vi "Set BlowerHeater.vi"(7 "Blower/Heater":T1, 8 "error in (no error)":errorcluster, 10 "ON/OFF (OFF)":bool, 11 "cRIO-CO2 in":refnum<class "cRIO-CO2.lvclass">) -> (0 "error out":errorcluster, 3 "cRIO-CO2 out":refnum<class "cRIO-CO2.lvclass">)   [LabVIEW 2015, in "cRIO-Carbondioxide.lvlib" / "cRIO-CO2.lvlib" / "cRIO-CO2.lvclass"]
uses:
  cRIO-CO2.lvclass
  Blowers Heaters Enumerator.ctl
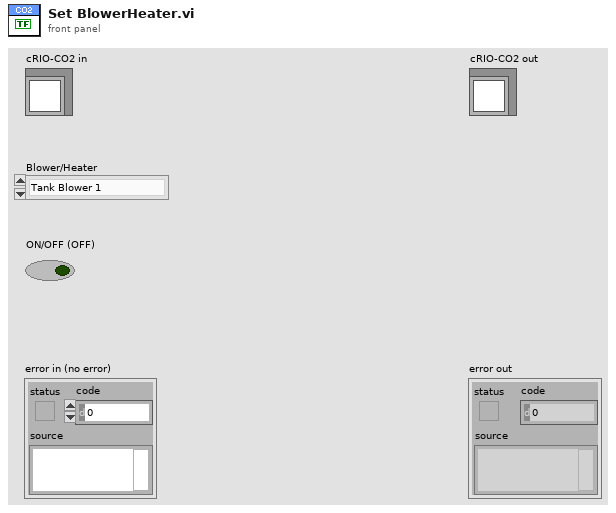
[diagram p1: front panel]
types:
  T1 = typedef "cRIO-Carbondioxide.lvlib/cRIO-CO2.lvlib/cRIO-CO2.lvclass/Blowers Heaters Enumerator.ctl" = enum16{"Tank Blower 1", "Tank Blower 2", "Tank Blower 3", "Tank Blower 4", "Syringe Blower", "Syringe Heater", "Piston Heater", "Undefined"}
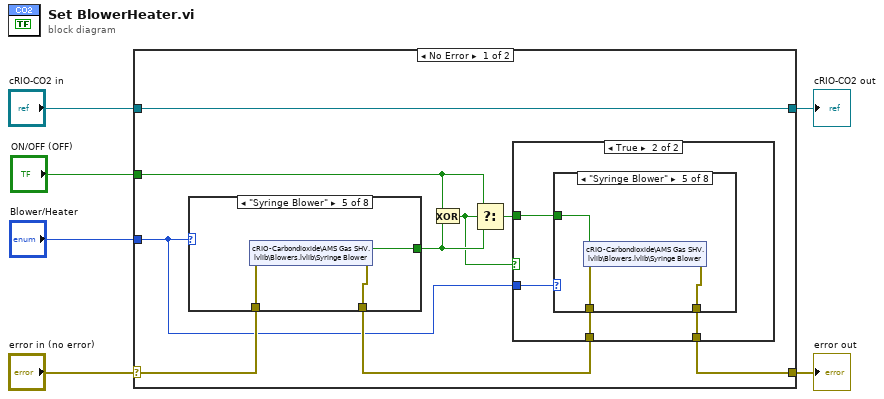
[diagram p0: block diagram]
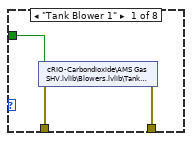
[diagram p3: hidden frame]
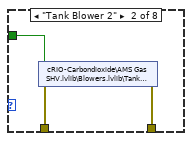
[diagram p4: hidden frame]
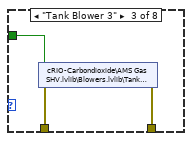
[diagram p5: hidden frame]
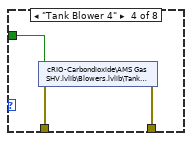
[diagram p6: hidden frame]
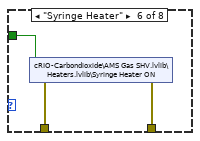
[diagram p7: hidden frame]
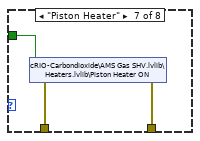
[diagram p8: hidden frame]
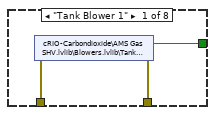
[diagram p10: hidden frame]
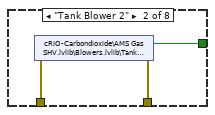
[diagram p11: hidden frame]
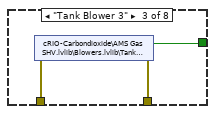
[diagram p12: hidden frame]
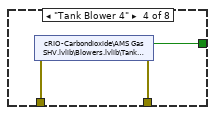
[diagram p13: hidden frame]
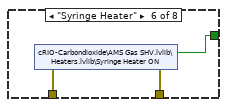
[diagram p14: hidden frame]
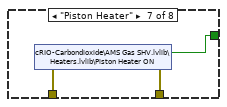
[diagram p15: hidden frame]
diagram:
  n1 = case shown="No Error" "error in (no error)" {
    selector: "error in (no error)" -> [w14 w66]
    tunnel: [w12 w66] -> w5
    tunnel: [w15 w65] -> w3
    tunnel: "cRIO-CO2 in" -> [w15 w65]
    tunnel: "Blower/Heater" -> [w11 _]
    tunnel: "ON/OFF (OFF)" -> [w9 _]
    frame No Error {
      n2 = case shown="\"Syringe Blower\"" w11 {
        tunnel: w14 -> [w45 w48 w51 w54 w57 w60 w63 w64]
        tunnel: [w44 w47 w50 w53 w56 w59 w62 w64] -> w13
        tunnel: [w43 w46 w49 w52 w55 w58 w61 _] -> w10
        frame "Tank Blower 1" {
          n3 = shared-variable "cRIO-Carbondioxide\\AMS Gas SHV.lvlib\\Blowers.lvlib\\Tank Blower 1"(error in=w45) -> (w43:bool, error out=w44:errorcluster)
        }
        frame "Tank Blower 2" {
          n4 = shared-variable "cRIO-Carbondioxide\\AMS Gas SHV.lvlib\\Blowers.lvlib\\Tank Blower 2"(error in=w48) -> (w46:bool, error out=w47:errorcluster)
        }
        frame "Tank Blower 3" {
          n5 = shared-variable "cRIO-Carbondioxide\\AMS Gas SHV.lvlib\\Blowers.lvlib\\Tank Blower 3"(error in=w51) -> (w49:bool, error out=w50:errorcluster)
        }
        frame "Tank Blower 4" {
          n6 = shared-variable "cRIO-Carbondioxide\\AMS Gas SHV.lvlib\\Blowers.lvlib\\Tank Blower 4"(error in=w54) -> (w52:bool, error out=w53:errorcluster)
        }
        frame "Syringe Blower" {
          n7 = shared-variable "cRIO-Carbondioxide\\AMS Gas SHV.lvlib\\Blowers.lvlib\\Syringe Blower"(error in=w57) -> (w55:bool, error out=w56:errorcluster)
        }
        frame "Syringe Heater" {
          n8 = shared-variable "cRIO-Carbondioxide\\AMS Gas SHV.lvlib\\Heaters.lvlib\\Syringe Heater ON"(error in=w60) -> (w58:bool, error out=w59:errorcluster)
        }
        frame "Piston Heater" {
          n9 = shared-variable "cRIO-Carbondioxide\\AMS Gas SHV.lvlib\\Heaters.lvlib\\Piston Heater ON"(error in=w63) -> (w61:bool, error out=w62:errorcluster)
        }
        frame "Undefined" {
        }
      }
      n10 = Exclusive Or(1:w10, 2:w9) -> (0:w7:bool)
      n11 = Select(t=w9, s=w7, f=w10) -> (s? t:f=w8:bool)
      n12 = case shown="True" w7 {
        tunnel: w13 -> [w16 w20]
        tunnel: [w16 w19] -> w12
        tunnel: w11 -> [_ w18]
        tunnel: w8 -> [_ w17]
        frame False {
        }
        frame True {
          n13 = case shown="\"Syringe Blower\"" w18 {
            tunnel: w20 -> [w23 w26 w29 w32 w35 w38 w41 w42]
            tunnel: [w22 w25 w28 w31 w34 w37 w40 w42] -> w19
            tunnel: w17 -> [w21 w24 w27 w30 w33 w36 w39 _]
            frame "Tank Blower 1" {
              n14 = shared-variable "cRIO-Carbondioxide\\AMS Gas SHV.lvlib\\Blowers.lvlib\\Tank Blower 1"(w21, error in=w23) -> (error out=w22:errorcluster)
            }
            frame "Tank Blower 2" {
              n15 = shared-variable "cRIO-Carbondioxide\\AMS Gas SHV.lvlib\\Blowers.lvlib\\Tank Blower 2"(w24, error in=w26) -> (error out=w25:errorcluster)
            }
            frame "Tank Blower 3" {
              n16 = shared-variable "cRIO-Carbondioxide\\AMS Gas SHV.lvlib\\Blowers.lvlib\\Tank Blower 3"(w27, error in=w29) -> (error out=w28:errorcluster)
            }
            frame "Tank Blower 4" {
              n17 = shared-variable "cRIO-Carbondioxide\\AMS Gas SHV.lvlib\\Blowers.lvlib\\Tank Blower 4"(w30, error in=w32) -> (error out=w31:errorcluster)
            }
            frame "Syringe Blower" {
              n18 = shared-variable "cRIO-Carbondioxide\\AMS Gas SHV.lvlib\\Blowers.lvlib\\Syringe Blower"(w33, error in=w35) -> (error out=w34:errorcluster)
            }
            frame "Syringe Heater" {
              n19 = shared-variable "cRIO-Carbondioxide\\AMS Gas SHV.lvlib\\Heaters.lvlib\\Syringe Heater ON"(w36, error in=w38) -> (error out=w37:errorcluster)
            }
            frame "Piston Heater" {
              n20 = shared-variable "cRIO-Carbondioxide\\AMS Gas SHV.lvlib\\Heaters.lvlib\\Piston Heater ON"(w39, error in=w41) -> (error out=w40:errorcluster)
            }
            frame "Undefined" {
            }
          }
        }
      }
    }
    frame Error {
    }
  }
  "error out" <- w5
  "cRIO-CO2 out" <- w3
